vi "TMCM351-goJog.vi"(4 "执行？":bool, 5 "错误输入":errorcluster caption="错误输入（无错误）", 6 "step in":i32, 7 "motor":u8(ring) items=["x", "y", "z"], 8 "com in":refnum<visa-resource-name>) -> (0 "错误输出":errorcluster, 3 "com out":refnum<visa-resource-name>)   [LabVIEW 2018]
uses:
  module_param.vi
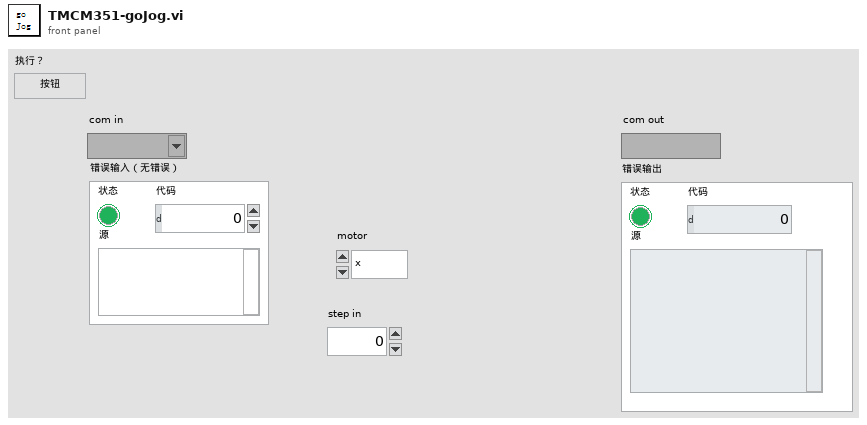
[diagram p1: front panel]
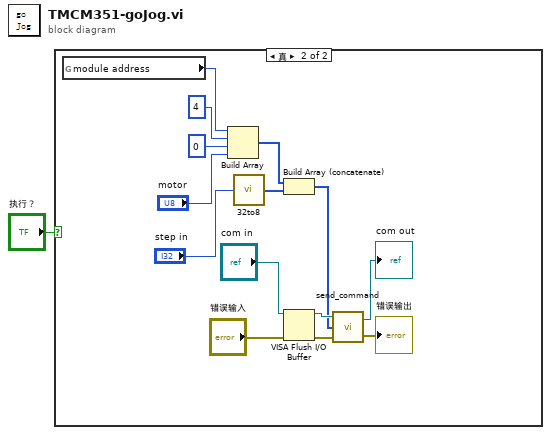
[diagram p0: block diagram]
diagram:
  n1 = case shown="真" "执行？" {
    frame False {
    }
    frame True {
      n2 = global read "module_param.vi" "module address"() -> (w14:u8)
      n3 = Build Array(w14, u8 4 ("元素"), u8 0, "motor") -> (w6:u8[])
      n4 = call "32to8.vi"("32data_in"="step in") -> ("8Array"=w5:u8[])
      n5 = Build Array (concatenate)(w6, w5) -> (w4:u8[])
      n6 = VISA Flush I/O Buffer(VISA resource name="com in", error in (no error)="错误输入") -> (VISA resource name out=w10:refnum<visa-resource-name>, error out=w9:errorcluster)  [unwired: 1 in]
      n7 = call "send_command.vi"("错误输入"=w9, 3:w4, "com in"=w10) -> ("错误输出"=→"错误输出":errorcluster, "com out"=→"com out":refnum<visa-resource-name>)
    }
  }
